vi "ConvertTimestamp.vi"(11 "Time Stamp":timestamp) -> (2 "Timestamp out":i64)   [LabVIEW 2017]
doc: "Converts a LabVIEW timestamp to a unix timestamp."
uses:
  <vilib>/Utility/miscctls.llb/LVDateTimeRec.ctl
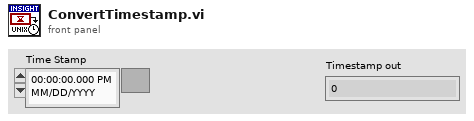
[diagram p1: front panel]
types:
  T1 = typedef "LVDateTimeRec.ctl" = cluster{"fractional second":dbl, "second":i32, "minute":i32, "hour":i32, "day of month":i32, "month":i32, "year":i32, "day of week":i32, "day of year":i32, "DST":i32}
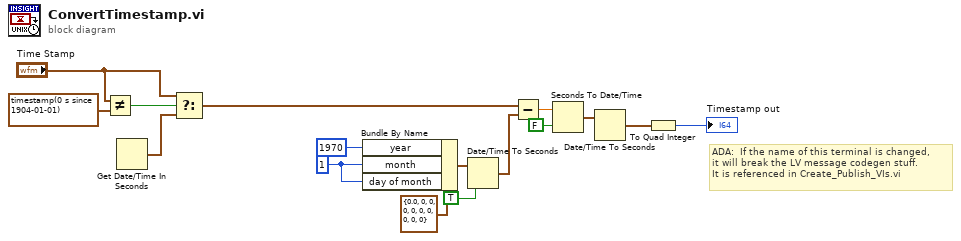
[diagram p0: block diagram]
diagram:
  w6 = 1 ("month")
  # "ADA:  If the name of this terminal is changed,\nit will break the LV message codegen stuff.\nIt is referenced in Create_Publish_VIs.vi"
  n1 = Not Equal?(x="Time Stamp", y=timestamp(0 s since 1904-01-01)) -> (x != y?=w14:bool)
  n2 = Get Date/Time In Seconds() -> (seconds since 1Jan1904=w3:timestamp)
  n3 = Select(t="Time Stamp", s=w14, f=w3) -> (s? t:f=w1:timestamp)
  n4 = Bundle By Name(cluster=T1 {"fractional second"=0.0, "second"=0, "minute"=0, "hour"=0, "day of month"=0, "month"=0, "year"=0, "day of week"=0, "day of year"=0, "DST"=0} ("date time rec"), "year"=1970, "month"=w6, "day of month"=w6) -> (w8:T1)
  n5 = Date/Time To Seconds(1:TRUE ("is UTC (F)"), 2:w8) -> (0:w10:timestamp)
  n6 = Subtract(x=w1, y=w10) -> (x-y=w11:dbl)
  n7 = Seconds To Date/Time(time stamp (now)=w11, to UTC (F)=FALSE) -> (date time rec=w12:T1)
  n8 = Date/Time To Seconds(2:w12) -> (0:w13:timestamp)  [unwired: 1 in]
  n9 = To Quad Integer(1:w13) -> (0:→"Timestamp out":i64)
